vi "Scan_Time.vi"(1 "时间差(ms)":dbl) -> (0 "时间字符串":string)   [LabVIEW 2020]
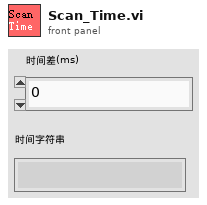
[diagram p1: front panel]
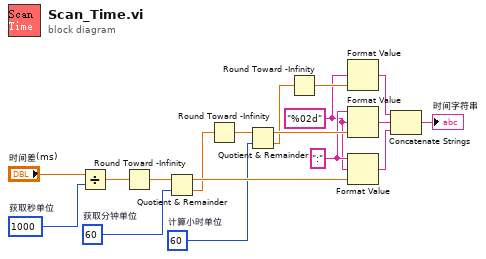
[diagram p0: block diagram]
diagram:
  w3 = "%02d"
  w4 = ":"
  w7 = 60  # 计算小时单位
  w6 = 60  # 获取分钟单位
  w5 = 1000  # 获取秒单位
  n1 = Divide(x="时间差(ms)", y=w5) -> (x/y=w9:dbl)
  n2 = Round Toward -Infinity(1:w9) -> (0:w8:dbl)
  n3 = Quotient & Remainder(x=w8, y=w6) -> (x-y*floor(x/y)=w13:dbl, floor(x/y)=w10:dbl)
  n4 = Round Toward -Infinity(1:w10) -> (0:w11:dbl)
  n5 = Quotient & Remainder(x=w11, y=w7) -> (x-y*floor(x/y)=w14:dbl, floor(x/y)=w12:dbl)
  n6 = Round Toward -Infinity(1:w12) -> (0:w15:dbl)
  n7 = Format Value(format string=w3, value (0)=w15) -> (output string=w16:string)  [unwired: 1 in]
  n8 = Format Value(string ("")=w4, format string=w3, value (0)=w14) -> (output string=w17:string)
  n9 = Format Value(string ("")=w4, format string=w3, value (0)=w13) -> (output string=w18:string)
  n10 = Concatenate Strings(w16, w17, w18) -> (→"时间字符串":string)
